vi "RLcmd Global.vi"() -> ()   [LabVIEW 2014]
panel:
  out "RLcmd Global":dbl
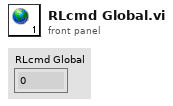
[diagram p1: front panel]
diagram:
